vi "Find Tags.vi"(11 "Package":refnum<class "Package.lvclass">) -> (3 "Tags Front Matter":string)   [LabVIEW 2020]
doc: "This method loads the VIPMTag file on first call and uses it to find keywords in the Display Name and Description. When a keyword is found the cooresponding Tag is added to the Tag list."
uses:
  Libraries/Packages/Package_class/Package.lvclass
  Libraries/Packages/Package_class/Package.lvclass/Package.ctl
  Libraries/Packages/Package Version_class/Package Version.lvclass/Package Version.ctl
  Libraries/Packages/Package Version_class/Read Author.vi
  Libraries/Packages/Package Version_class/Read Dependencies.vi
  Libraries/Packages/Package Version_class/Read Description.vi
  Libraries/Packages/Package Version_class/Read DisplayName.vi
  Libraries/Packages/Package Version_class/Read Name.vi
  Libraries/Packages/Package Version_class/Read Release Notes.vi
  Libraries/Packages/Package Version_class/Read RepoName.vi
  Libraries/Packages/Package Version_class/Read Vendor.vi
  Libraries/Packages/Package_class/Read DisplayName.vi
  Libraries/Packages/Package_class/Read Name.vi
  Libraries/Packages/Package_class/Read RepoName.vi
  Libraries/Packages/Package_class/Read Versions.vi
  Libraries/Packages/Package Version_class/Package Version.lvclass
  <vilib>/Utility/file.llb/Read Delimited Spreadsheet (string).vi
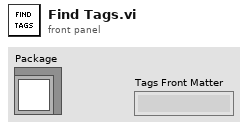
[diagram p1: front panel]
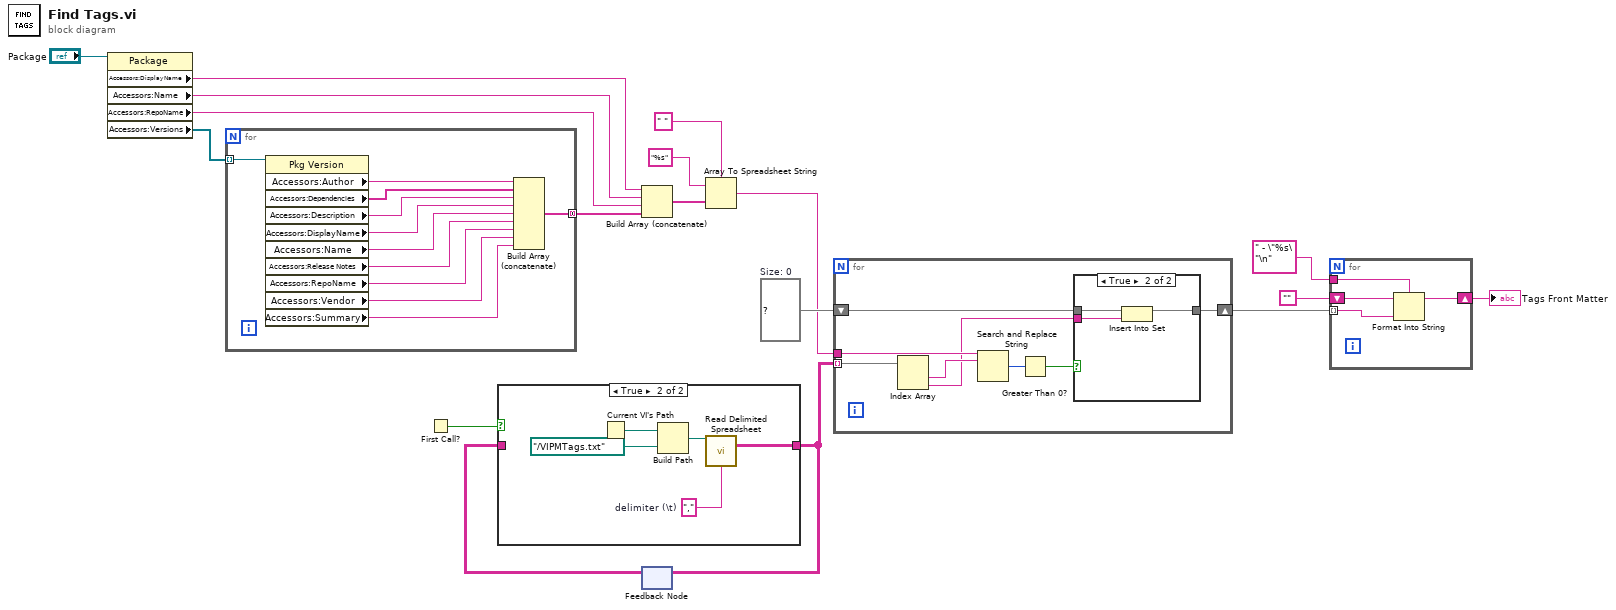
[diagram p0: block diagram]
diagram:
  w15 = set{string} {}  # Size: 0
  n1 = property class="Package"(reference="Package") -> ("Accessors:DisplayName"=w8:string, "Accessors:Name"=w7:string, "Accessors:RepoName"=w6:string, "Accessors:Versions"=w9:refnum<class "Package Version.lvclass">[])  [unwired: 1 in, 2 out]
  n2 = for {
    tunnel: w9 -> [w29] mode=indexing
    tunnel: [w20] -> w5 mode=concatenating
    n3 = property class="Pkg Version"(reference=w29) -> ("Accessors:Author"=w28:string, "Accessors:Dependencies"=w27:string[], "Accessors:Description"=w26:string, "Accessors:DisplayName"=w25:string, "Accessors:Name"=w24:string, "Accessors:Release Notes"=w23:string, "Accessors:RepoName"=w22:string, "Accessors:Vendor"=w21:string, "Accessors:Summary"=w19:string)  [unwired: 1 in, 2 out]
    n4 = Build Array (concatenate)(w28, w27, w26, w25, w24, w23, w22, w21, w19) -> (w20:string[])
  }
  n5 = First Call?() -> (First Call?: T/F=w18:bool)
  n6 = Build Array (concatenate)(w8, w7, w6, w5) -> (w4:string[])
  n7 = feedback #1() -> (w16:string[][])  [unwired: 1 in]
  n8 = case shown="True" w18 {
    tunnel: [w30 w31] -> w17
    tunnel: w16 -> [w30 _]
    frame False {
    }
    frame True {
      w32 = ","  # delimiter (\t)
      n9 = Current VI's Path() -> (path=w35:path)
      n10 = Build Path(base path=w35, name or relative path=path "../VIPMTags.txt") -> (appended path=w33:path)
      n11 = call-poly <vilib>:"Read Delimited Spreadsheet.vi"("file path (dialog if empty)"=w33, "delimiter (\\t)"=w32) -> ("all rows"=w31:string[][])  [unwired: 8 in, 5 out]
    }
  }
  n12 = feedback-in #1(w17) -> ()
  n13 = Array To Spreadsheet String(delimiter (Tab)=" ", array=w4, 3:"%s") -> (spreadsheet string=w2:string)
  n14 = for {
    tunnel: w2 -> [w43]
    tunnel: w17 -> [w41] mode=indexing
    shift-right: [w37] -> w14
    shift-left: w15 -> [w36]
    n15 = Index Array(array=w41) -> (element #1=w40:string, element #2=w39:string)  [unwired: 2 in]
    n16 = Search and Replace String(input string=w43, search string=w40) -> (number of replacements=w42:i32)  [unwired: 6 in, 3 out]
    n17 = Greater Than 0?(x=w42) -> (x > 0?=w38:bool)
    n18 = case shown="True" w38 {
      tunnel: w39 -> [_ w47]
      tunnel: [w44 w46] -> w37
      tunnel: w36 -> [w44 w45]
      frame False {
      }
      frame True {
        n19 = Insert Into Set(10:w47, 11:w45) -> (3:w46:set{string})  [unwired: 1 out]
      }
    }
  }
  n20 = for {
    tunnel: w14 -> [w51] mode=indexing
    shift-right: [w49] -> w11
    shift-left: "" -> [w50]
    tunnel: " - \"%s\"\n" -> [w48]
    n21 = Format Into String(format string=w48, initial string=w50, w51) -> (resulting string=w49:string)  [unwired: 1 in, 1 out]
  }
  "Tags Front Matter" <- w11
